vi "Merge Builds.vi"(7 "Offer remove other builds after merge? (False)":bool, 8 "error in":errorcluster, 10 "wildcard serach key for exe file (e.g.: power?cal*.exe)":string="power?cal*.exe", 11 "Destination Path":path) -> (0 "error out":errorcluster, 3 "other builds to remove":path[](array[path]))   [LabVIEW 2020]
doc: "This VI will look for builds of the same version number and copies the other builds' EXE files to this build. This VI should be called only from the main main build with all drivers or it may do some crazy stuff. It will optionally offer removal of the other builds after merge."
uses:
  <vilib>/regexp/Match Regular Expression.xnode
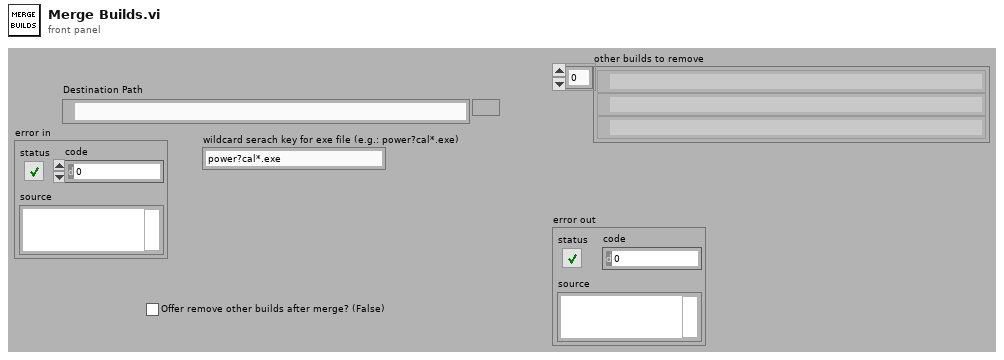
[diagram p1: front panel]
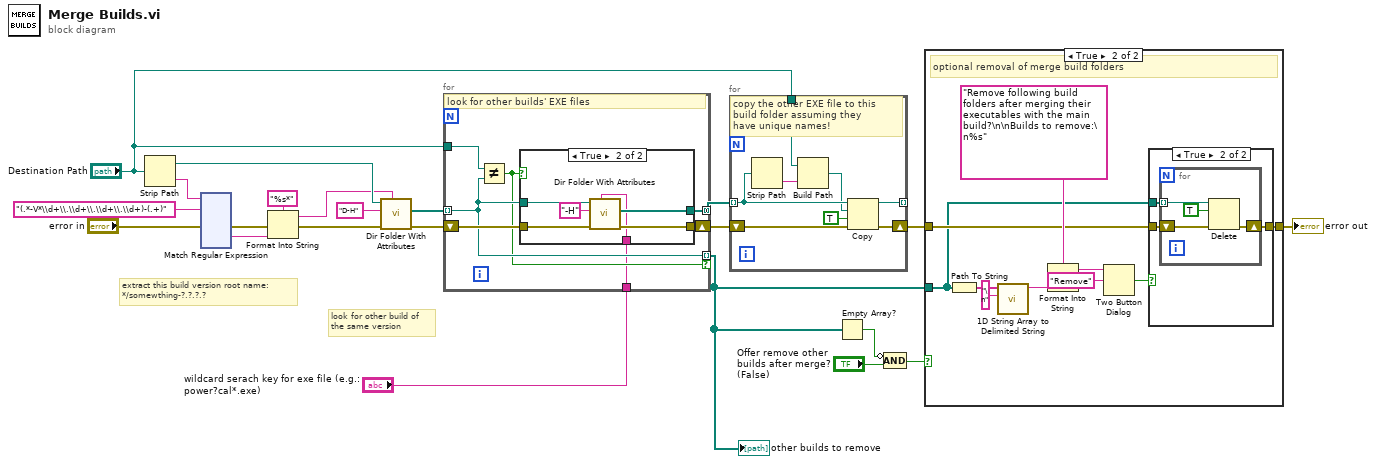
[diagram p0: block diagram]
diagram:
  # "look for other build of\nthe same version"
  # "extract this build version root name:\n*/somewthing-?.?.?.?"
  n1 = Strip Path(path="Destination Path") -> (stripped path=w14:path, name=w22:string)
  n2 = xnode "Match Regular Expression"("input string"=w22, "regular expression"="(.*-V*\\d+\\.\\d+\\.\\d+\\.\\d+)-(.+)", "error in"="error in") -> ("error out"=w20:errorcluster, "submatch 1"=w16:string)  [unwired: 3 in, 5 out]
  n3 = Format Into String(format string="%s*", error in=w20, w16) -> (resulting string=w13:string, error out=w19:errorcluster)  [unwired: 1 in]
  n4 = call "Dir Folder With Attributes.vi"("wildcard serach key (*)"=w13, "error in (no error)"=w19, "\"DIR /A:?\" attribute(s) (default: -H)"="D-H" ("\"DIR /A:?\" attribute(s) (default: -H)"), "folder"=w14) -> ("error out"=w12:errorcluster, "file/folder paths"=w15:path[])  [unwired: 5 in, 1 out]
  n5 = for {
    tunnel: "Destination Path" -> [w29]
    tunnel: w15 -> [w25] mode=indexing
    shift-right: [w27] -> w10
    shift-left: w12 -> [w28]
    tunnel: [w26] -> w9 mode=concatenating
    tunnel: [w25] -> w6 mode=indexing if=w24
    tunnel: "wildcard serach key for exe file (e.g.: power?cal*.exe)" -> [w23]
    # "look for other builds' EXE files"
    n6 = Not Equal?(x=w29, y=w25) -> (x != y?=w24:bool)
    n7 = case shown="True" w24 {
      tunnel: w28 -> [w30 w36]
      tunnel: w25 -> [_ w32]
      tunnel: [w30 w35] -> w27
      tunnel: [_ w33] -> w26
      tunnel: w23 -> [_ w31]
      frame False {
      }
      frame True {
        n8 = call "Dir Folder With Attributes.vi"("wildcard serach key (*)"=w31, "error in (no error)"=w36, "\"DIR /A:?\" attribute(s) (default: -H)"="-H" ("\"DIR /A:?\" attribute(s) (default: -H)"), "folder"=w32) -> ("error out"=w35:errorcluster, "file/folder paths"=w33:path[])  [unwired: 5 in, 1 out]
      }
    }
  }
  "other builds to remove" <- w6
  n9 = for {
    shift-right: [w38] -> w7
    shift-left: w10 -> [w44]
    tunnel: w9 -> [w41] mode=indexing
    tunnel: "Destination Path" -> [w42]
    tunnel: [w37] -> _ mode=indexing
    # "copy the other EXE file to this\nbuild folder assuming they\nhave unique names!"
    n10 = Strip Path(path=w41) -> (name=w43:string)  [unwired: 1 out]
    n11 = Build Path(base path=w42, name or relative path=w43) -> (appended path=w40:path)
    n12 = Copy(8:w44, 9:TRUE ("overwrite (F)"), 10:w40, 11:w41) -> (0:w38:errorcluster, 3:w37:path)  [unwired: 1 in, 1 out]
  }
  n13 = Empty Array?(array=w6) -> (empty?=w3:bool)
  n14 = Compound Arithmetic op=AND(invert w3, "Offer remove other builds after merge? (False)") -> (w5:bool)
  n15 = case shown="True" w5 {
    tunnel: w7 -> [w45 w49]
    tunnel: w6 -> [_ w48]
    tunnel: [w45 w47] -> w2
    frame False {
    }
    frame True {
      # "optional removal of merge build folders"
      n16 = Path To String(path=w48) -> (string=w55:string[])
      n17 = call <vilib>:"1D String Array to Delimited String.vi"("delimiter"="\n", "string array"=w55) -> ("delimited string"=w53:string)  [unwired: 9 in]
      n18 = Format Into String(format string="Remove following build folders after merging their executables with the main build?\n\nBuilds to remove:\n%s", w53) -> (resulting string=w51:string)  [unwired: 2 in, 1 out]
      n19 = Two Button Dialog(message=w51, 2:"Remove" ("T button name (\"OK\")")) -> (T button?=w46:bool)  [unwired: 1 in]
      n20 = case shown="True" w46 {
        tunnel: w49 -> [w56 w59]
        tunnel: w48 -> [_ w58]
        tunnel: [w56 w57] -> w47
        frame False {
        }
        frame True {
          n21 = for {
            shift-right: [w62] -> w57
            shift-left: w59 -> [w63]
            tunnel: w58 -> [w60] mode=indexing
            n22 = Delete(path (use dialog)=w60, entire hierarchy (F)=TRUE, error in=w63) -> (error out=w62:errorcluster)  [unwired: 2 in, 2 out]
          }
        }
      }
    }
  }
  "error out" <- w2
